vi "Écrire Symbol_Suffix.vi"(8 "error in (no error)":errorcluster caption="entrée d'erreur (pas d'erreur)", 10 "Symbol_Suffix":string=".PA", 11 "Stock en entrée":refnum<class "Stock.lvclass">) -> (0 "error out":errorcluster caption="sortie d'erreur", 3 "Stock en sortie":refnum<class "Stock.lvclass">)   [LabVIEW 2012, in "Stock.lvclass"]
uses:
  Stock.lvclass
  Stock.lvclass/Stock.ctl
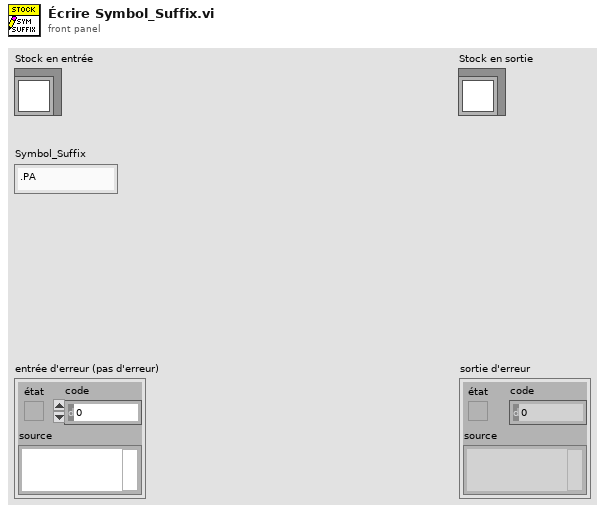
[diagram p1: front panel]
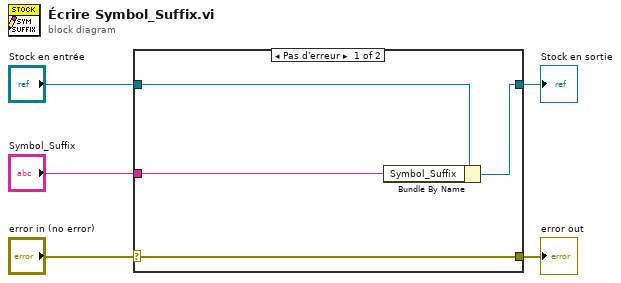
[diagram p0: block diagram]
diagram:
  n1 = case shown="Pas d'erreur" "error in (no error)" {
    selector: "error in (no error)" -> [w9 w10]
    tunnel: [w9 w10] -> w4
    tunnel: [w7 w11] -> w2
    tunnel: "Stock en entrée" -> [w8 w11]
    tunnel: "Symbol_Suffix" -> [w6 _]
    frame No Error {
      n2 = Bundle By Name(cluster=w8, "Symbol_Suffix"=w6) -> (w7:refnum<class "Stock.lvclass">)
    }
    frame Error {
    }
  }
  "error out" <- w4
  "Stock en sortie" <- w2
